vi "HP - Read group position.vi"(2 "error in":errorcluster, 3 "Group #":i8=1 min=1 max=6 step=1, 4 "Address / Port":i16=1 min=1 max=31 step=1) -> (0 "error out":errorcluster, 1 "Query the current position\nof group - read":dbl format="%.2f")   [LabVIEW 2014]
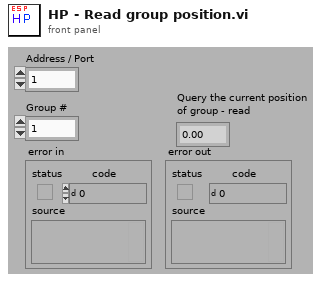
[diagram p1: front panel]
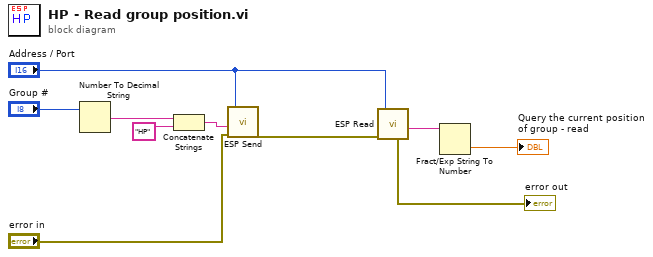
[diagram p0: block diagram]
diagram:
  n1 = Number To Decimal String(number="Group #") -> (decimal integer string=w9:string)  [unwired: 1 in]
  n2 = Concatenate Strings(w9, "HP" ("Substring")) -> (w7:string)
  n3 = call "ESP Send.vi"("Address / Port"="Address / Port", "Command String"=w7, "error in"="error in") -> ("error out"=w4:errorcluster)  [unwired: 5 in]
  n4 = call "ESP Read.vi"("Address / Port"="Address / Port", "error in"=w4) -> ("error out"=→"error out":errorcluster, "Response String"=w5:string)  [unwired: 5 in]
  n5 = Fract/Exp String To Number(string=w5) -> (number=→"Query the current position\nof group - read":dbl)  [unwired: 3 in, 1 out]
